vi "Read B.vi"(8 "error in (no error)":errorcluster, 11 "Arithmetic Operations in":refnum<class "Arithmetic Operations.lvclass">) -> (0 "error out":errorcluster, 2 "B":dbl, 3 "Arithmetic Operations out":refnum<class "Arithmetic Operations.lvclass">)   [LabVIEW 2020, in "Arithmetic Operations.lvclass"]
uses:
  Arithmetic Operations.lvclass
  Arithmetic Operations.lvclass/Arithmetic Operations.ctl
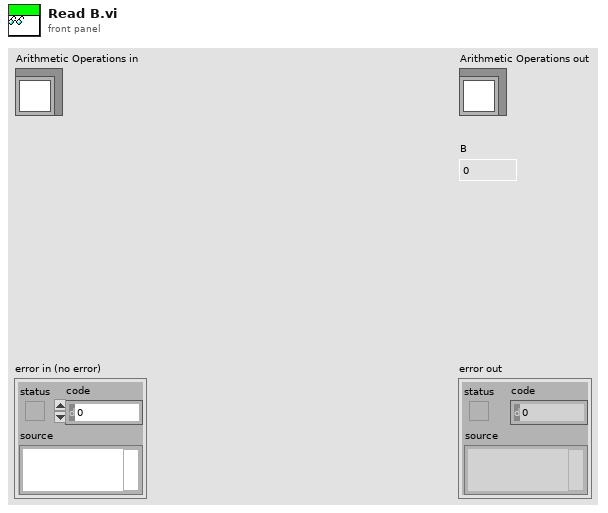
[diagram p1: front panel]
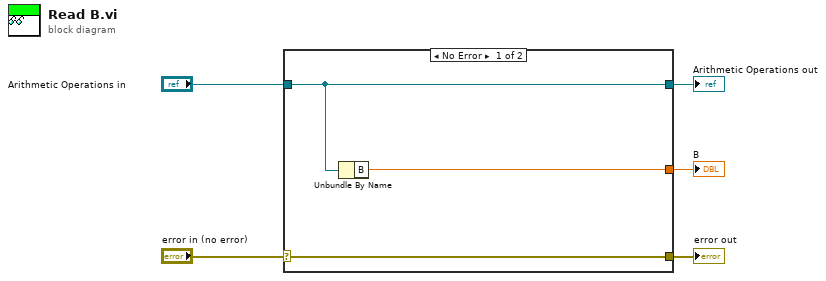
[diagram p0: block diagram]
diagram:
  n1 = case shown="No Error" "error in (no error)" {
    selector: "error in (no error)" -> [w8 w9]
    tunnel: [w8 w9] -> w4
    tunnel: [w7 w10] -> w2
    tunnel: "Arithmetic Operations in" -> [w7 w10]
    tunnel: [w6 _] -> w1
    frame No Error {
      n2 = Unbundle By Name(w7) -> ("B"=w6:dbl)
    }
    frame Error {
    }
  }
  "error out" <- w4
  "Arithmetic Operations out" <- w2
  "B" <- w1
